vi "GetItemstoGrade.vi"(0 "Paths":T2) -> ()   [LabVIEW 2012]
uses:
  <userlib>/BotSpeak/Devices/EvalRIO/HTTPServer/PathsGlobal.ctl
panel:
  out "status":string
  out "dropBox":string
  out "last":T1
  in  "Download":bool
  in  "Done":bool
  in  "Btns":T1
  in  "Books":i32[](listbox)
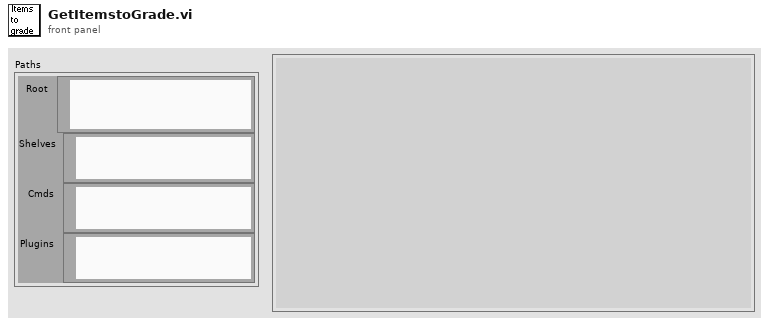
[diagram p1: front panel]
types:
  T1 = cluster{"book":bool, "user":bool, "Filename":bool}
  T2 = typedef "PathsGlobal.ctl" = cluster{"Root":path, "Shelves":path, "Cmds":path, "Plugins":path}
  T3 = cluster{"book names":string[], "authors":string[], "filename":string[]}
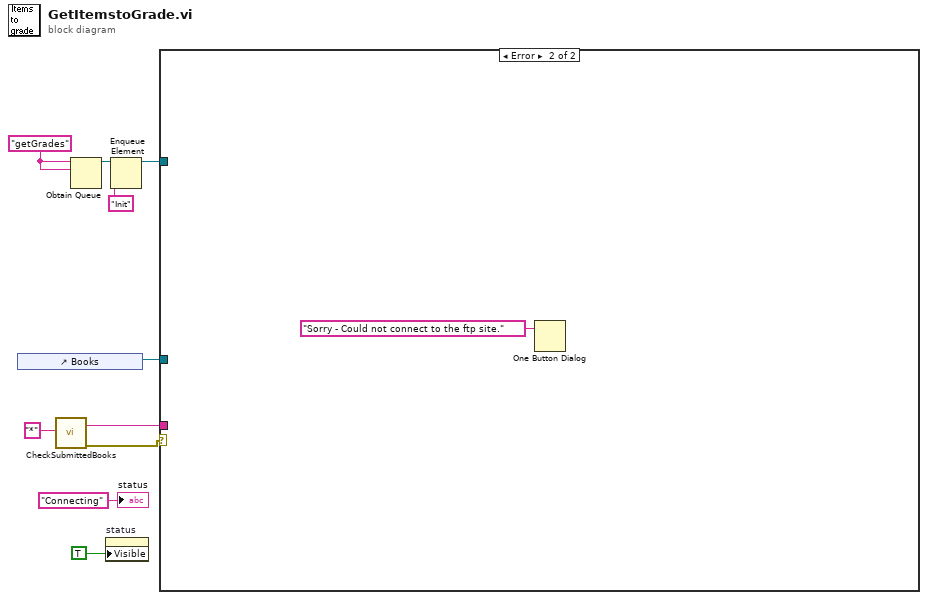
[diagram p0: block diagram]
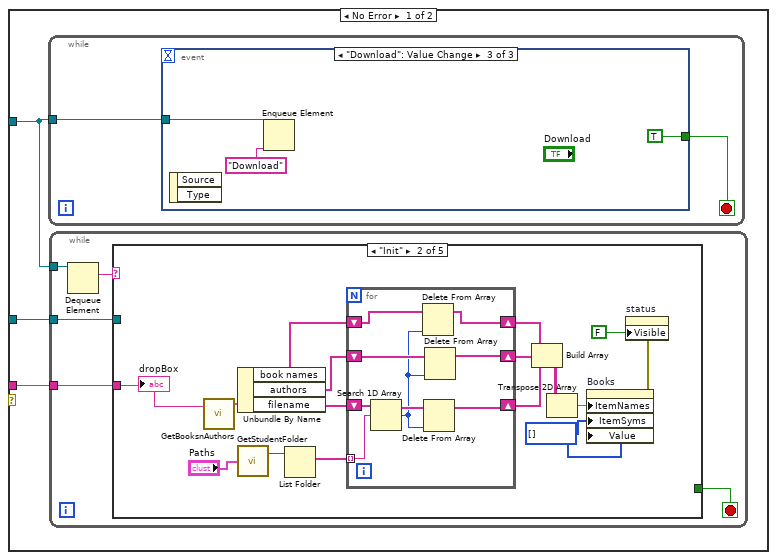
[diagram p2: hidden frame]
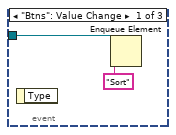
[diagram p3: hidden frame]
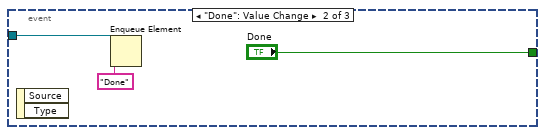
[diagram p4: hidden frame]
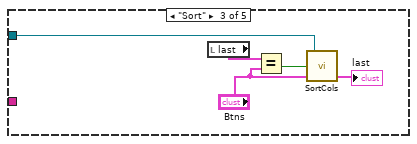
[diagram p6: hidden frame]
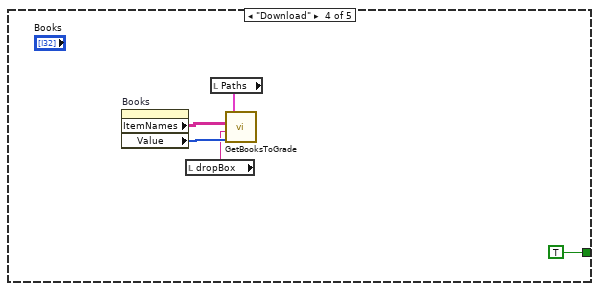
[diagram p7: hidden frame]
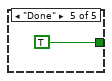
[diagram p8: hidden frame]
diagram:
  w8 = "getGrades" ("name (unnamed)")
  n1 = control-ref of="Books"() -> (w7:refnum<vi>)
  n2 = call <userlib>:"CheckSubmittedBooks.vi"("Username"="*") -> ("error out"=w2:errorcluster, "dropBox"=w1:string)  [unwired: 2 in, 4 out]
  n3 = Obtain Queue(name (unnamed)=w8, element data type=w8) -> (queue out=w10:refnum<queue>)  [unwired: 3 in, 2 out]
  n4 = property on="status" class="Str"("Visible"=TRUE) -> ()  [unwired: 2 in, 2 out]
  n5 = Enqueue Element(queue=w10, element="Init") -> (queue out=w6:refnum<queue>)  [unwired: 1 in, 3 out]
  n6 = case shown="Error" w2 {
    tunnel: w7 -> [w13 _]
    tunnel: w6 -> [w12 _]
    tunnel: w1 -> [w11 _]
    frame No Error {
      n7 = while {
        tunnel: w12 -> [w15]
        stop <- w14 stop-if-true
        n8 = event shown="[2] \"Download\": Value Change" {
          selector: _ -> [_ _ _]
          dyn-events: _ -> [_ _ _]
          timeout: _ -> [_ _ _]
          tunnel: w15 -> [w16 w19 w22]
          tunnel: [_ "Done" TRUE ("Done")] -> w14
          event "Btns": Value Change {
            n9 = event-data() -> ()  [unwired: 2 out]
            n10 = Enqueue Element(queue=w16, element="Sort") -> ()  [unwired: 1 in, 4 out]
          }
          event "Done": Value Change {
            n11 = event-data() -> ()  [unwired: 3 out]
            n12 = Enqueue Element(queue=w19, element="Done") -> ()  [unwired: 1 in, 4 out]
          }
          event "Download": Value Change {
            n13 = event-data() -> ()  [unwired: 3 out]
            n14 = Enqueue Element(queue=w22, element="Download") -> ()  [unwired: 1 in, 4 out]
          }
        }
      }
      n15 = while {
        tunnel: w12 -> [w28]
        tunnel: w13 -> [w26]
        tunnel: w11 -> [w24]
        stop <- w25 stop-if-true
        n16 = Dequeue Element(queue=w28) -> (element=w27:string)  [unwired: 1 in, 4 out]
        n17 = case shown="\"Init\"" w27 {
          tunnel: w26 -> [_ _ w57 _ _]
          tunnel: [_ _ _ TRUE TRUE] -> w25
          tunnel: w24 -> [_ w29 _ _ _]
          frame Default {
          }
          frame "Init" {
            w32 = i32[] [] ("Item Symbols")
            n18 = call <userlib>:"GetBooksnAuthors.vi"("reply string"=w29) -> ("Server Info"=w41:T3)  [unwired: 3 out]
            n19 = Unbundle By Name(w41) -> ("book names"=w39:string[], "authors"=w38:string[], "filename"=w43:string[])
            n20 = call <userlib>:"GetStudentFolder.vi"("Paths"="Paths") -> ("Student"=w42:path)  [unwired: 1 out]
            n21 = List Folder(path=w42) -> (filenames=w44:string[])  [unwired: 1 in, 5 out]
            n22 = for {
              shift-right: [w50] -> w35
              shift-left: w43 -> [w51]
              tunnel: w44 -> [w52] mode=indexing
              shift-right: [w48] -> w37
              shift-left: w39 -> [w49]
              shift-right: [w46] -> w36
              shift-left: w38 -> [w47]
              n23 = Search 1D Array(1D array=w51, element=w52) -> (index of element=w45:i32)  [unwired: 1 out]
              n24 = Delete From Array(array=w49, index=w45) -> (array with subset deleted=w48:string[])  [unwired: 1 in, 1 out]
              n25 = Delete From Array(array=w51, index=w45) -> (array with subset deleted=w50:string[])  [unwired: 1 in, 1 out]
              n26 = Delete From Array(array=w47, index=w45) -> (array with subset deleted=w46:string[])  [unwired: 1 in, 1 out]
            }
            n27 = Build Array(w37, w36, w35) -> (w34:string[][])
            n28 = Transpose 2D Array(2D array=w34) -> (transposed array=w33:string[][])
            n29 = property on="Books" class="MCListbox (strict)"("ItemNames"=w33, "ItemSyms"=w32, "Value"=w32) -> (error out=w30:errorcluster)  [unwired: 2 in, 1 out]
            n30 = property on="status" class="Str"(error in=w30, "Visible"=FALSE) -> ()  [unwired: 1 in, 2 out]
            "dropBox" <- w29
          }
          frame "Sort" {
            n31 = local read "last"() -> (w55:T1)
            n32 = Equal?(x=w55, y="Btns") -> (x = y?=w56:bool)
            n33 = call <userlib>:"SortCols.vi"("Btns"="Btns", "flip?"=w56, "Books"=w57) -> ("Btns out"=→"last":T1)  [unwired: 2 out]
          }
          frame "Download" {
            n34 = property on="Books" class="MCListbox (strict)"() -> ("ItemNames"=w62:string[][], "Value"=w61:i32[])  [unwired: 2 in, 2 out]
            n35 = local read "dropBox"() -> (w58:string)
            n36 = local read "Paths"() -> (w60:T2)
            n37 = call <userlib>:"GetBooksToGrade.vi"("Value"=w61, "dropBox"=w58, "ItemNames"=w62, "Paths"=w60) -> ()  [unwired: 3 out]
          }
          frame "Done" {
          }
        }
      }
    }
    frame Error {
      n38 = One Button Dialog(message="Sorry - Could not connect to the ftp site.") -> ()  [unwired: 2 out]
    }
  }
  "status" <- "Connecting" ("status")
